vi "pointListToLVPlot.vi"(1 "XY[N,d]":dbl[][](array[numeric])) -> (0 "LV plot":cluster{dbl[], dbl[]})   [LabVIEW 2017]
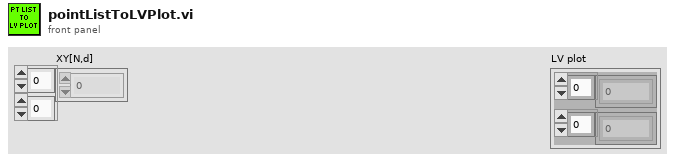
[diagram p1: front panel]
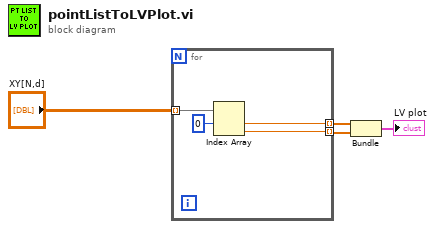
[diagram p0: block diagram]
diagram:
  n1 = for {
    tunnel: "XY[N,d]" -> [w8] mode=indexing
    tunnel: [w6] -> w4 mode=indexing
    tunnel: [w5] -> w3 mode=indexing
    n2 = Index Array(array=w8, index #1=0 ("index")) -> (element #1=w6:dbl, element #2=w5:dbl)  [unwired: 1 in]
  }
  n3 = Bundle(w4, w3) -> (→"LV plot":cluster{dbl[], dbl[]})  [unwired: 1 in]
